vi "Linear to dB.vi"(0 "linear value":dbl format="%.2f", 1 "attenuation?":bool=TRUE) -> (2 "dB value":dbl format="%.2f")   [LabVIEW 2020, in "NI_AAL_Filter.lvlib"]
uses:
  <vilib>/Analysis/NI_AAL_Filter.lvlib
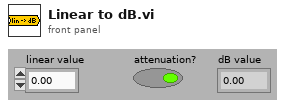
[diagram p1: front panel]
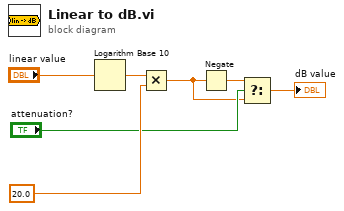
[diagram p0: block diagram]
diagram:
  n1 = Logarithm Base 10(1:"linear value") -> (0:w5:dbl)
  n2 = Multiply(x=w5, y=20.0) -> (x*y=w2:dbl)
  n3 = Negate(x=w2) -> (-x=w7:dbl)
  n4 = Select(t=w7, s="attenuation?", f=w2) -> (s? t:f=→"dB value":dbl)
